vi "GT Arc YZR.vi"(0 "cardNum":i16, 1 "radius":dbl, 2 "synVel":dbl, 3 "velEnd":dbl, 5 "crd":i16, 7 "y":i32, 9 "z":i32, 11 "error in (no error)":errorcluster caption="错误输入（无错误）", 12 "circleDir":i16, 13 "synAcc":dbl, 14 "fifo":i16) -> (4 "cardNum":i16, 15 "error out":errorcluster caption="错误输出")   [LabVIEW 2020, in "gts.lvlib"]
doc: "GT_API GT_ArcYZR(short cardNum,short crd,long y,long z,double radius,short circleDir,double synVel,double synAcc,double velEnd=0,short fifo=0);"
uses:
  gts.lvlib
  dll/32bit/multi_card/gts.dll
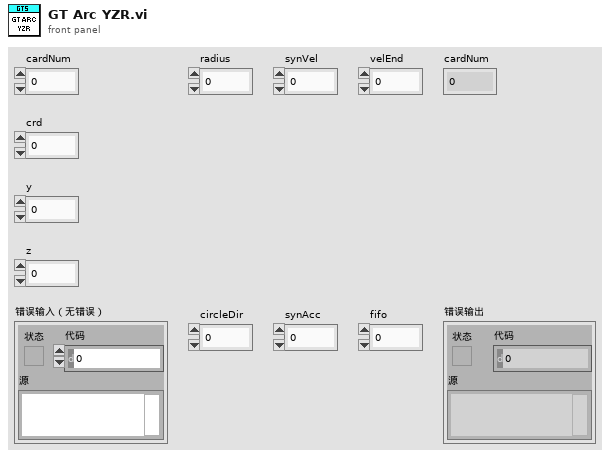
[diagram p1: front panel]
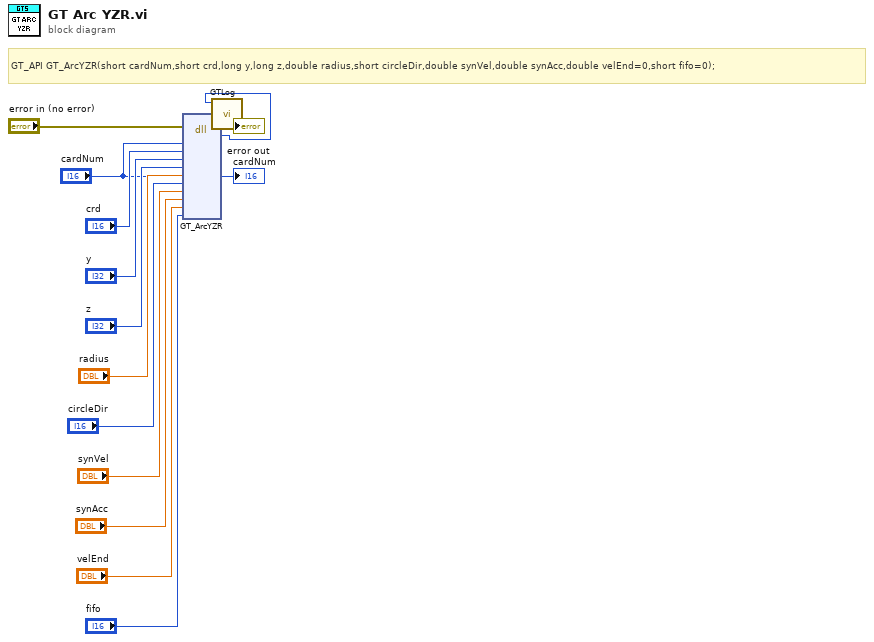
[diagram p0: block diagram]
diagram:
  # "GT_API GT_ArcYZR(short cardNum,short crd,long y,long z,double radius,short circleDir,double synVel,double synAcc,double velEnd=0,short fifo=0);"
  n1 = dll-call lib="D:/Git/GoogolCard/dll/32bit/multi_card/gts.dll" fn="GT_ArcYZR"(error in="error in (no error)", "cardNum"="cardNum", "crd"="crd", "y"="y", "z"="z", "radius"="radius", "circleDir"="circleDir", "synVel"="synVel", "synAcc"="synAcc", "velEnd"="velEnd", "fifo"="fifo") -> (error out=w4:errorcluster, w2:i16)  [unwired: 12 in, 1 out]
  n2 = call "GTLog.vi"("error in (no error)"=w4, "Numeric"=w2) -> ("error out"=→"error out":errorcluster)  [unwired: 9 in]
  "cardNum" <- "cardNum"
